vi "Property Node (SSH Client).vi"   [LabVIEW 2020, in "NI_SSH.lvlib"]
uses:
  <vilib>/net/SSH/NI_SSH.lvlib
  <vilib>/net/SSH/Client/Generic/Generic Client.lvclass
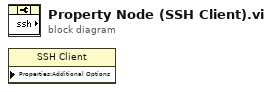
[diagram p0: block diagram]
diagram:
  n1 = property class="SSH Client" props=["Properties:Additional Options"]() -> ()  [unwired: 3 in, 2 out]
